vi "Value Pair Array Write.vi"(8 "error in (no error)":errorcluster, 9 "Value Pair Array":cluster{"Value":sgl, "Name":string}[](array[cluster]), 11 "3D Plot.lvclass in":refnum<class "3D Plot.lvclass">) -> (0 "error out":errorcluster, 3 "3D Plot.lvclass out":refnum<class "3D Plot.lvclass">)   [LabVIEW 2020, in "3D Plot.lvclass"]
uses:
  <vilib>/Math Plots/3D Math Plots/3D Plot/3D Plot/3D Plot.lvclass
  <vilib>/Math Plots/3D Math Plots/3D Plot/3D Plot/3D Plot.lvclass/3D Plot.ctl
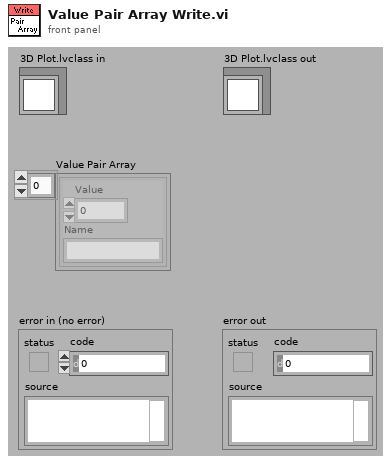
[diagram p1: front panel]
types:
  T1 = typedef "3D Plot.lvclass/Value Pair Property.ctl" = T2[]
  T2 = typedef "3D Plot.lvclass/Value Pair Cluster.ctl" = cluster{"Value Pair Array":cluster{"Value":sgl, "Name":string}[], "Show Tick":bool, "Show Grid":bool, " Label Mode":enum16{"Name", "Value", "None"}}
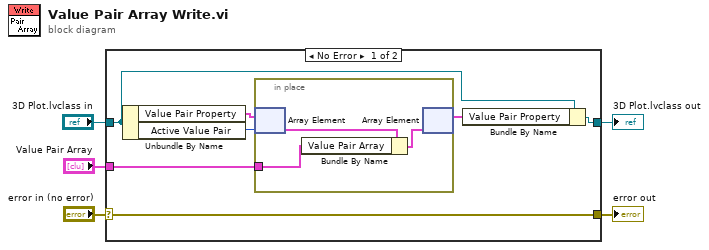
[diagram p0: block diagram]
diagram:
  n1 = case shown="No Error" "error in (no error)" {
    selector: "error in (no error)" -> [w10 w16]
    tunnel: "Value Pair Array" -> [w7 _]
    tunnel: "3D Plot.lvclass in" -> [w12 w17]
    tunnel: [w11 w17] -> w3
    tunnel: [w10 w16] -> w1
    frame No Error {
      n2 = Unbundle By Name(w12) -> ("Value Pair Property"=w9:T1, "Active Value Pair"=w8:enum16{"X-axis", "Y-axis", "Z-axis"})
      n3 = in-place {
        in-place-border: w7 -> [w14]
        n4 = in-place-array #1(w9, w8) -> (w15:T2)
        n5 = Bundle By Name(cluster=w15, "Value Pair Array"=w14) -> (w13:T2)
        n6 = in-place-array #1(w13) -> (w6:T1)  [unwired: 1 out]
      }
      n7 = Bundle By Name(cluster=w12, "Value Pair Property"=w6) -> (w11:refnum<class "3D Plot.lvclass">)
    }
    frame Error {
    }
  }
  "error out" <- w1
  "3D Plot.lvclass out" <- w3
